vi "Sweep_Speed.vi"() -> ()   [LabVIEW 2017]
panel:
  in  "speed":dbl
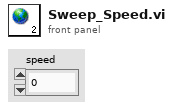
[diagram p1: front panel]
diagram:
